vi "Report.vi"(8 "error in":errorcluster, 9 "Received":path, 10 "Approved":path, 11 "Report Nothing in":refnum<class "Report Nothing.lvclass">) -> (0 "error out":errorcluster, 2 "Worked?":bool, 3 "Report Nothing out":refnum<class "Report Nothing.lvclass">)   [LabVIEW 2020, in "Approval Tests.lvlib" / "Report Nothing.lvclass"]
uses:
  Report Nothing.lvclass
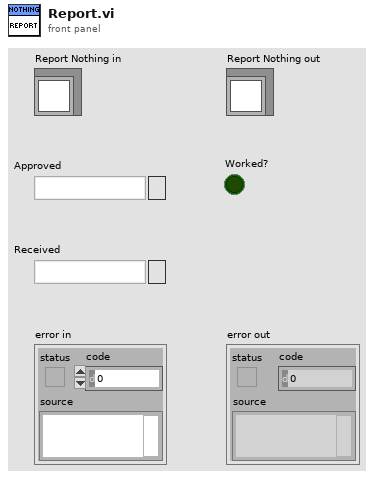
[diagram p1: front panel]
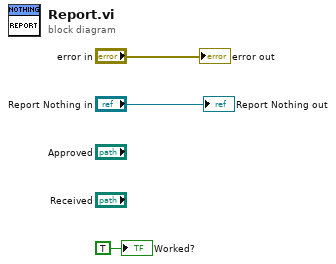
[diagram p0: block diagram]
diagram:
  "error out" <- "error in"
  "Report Nothing out" <- "Report Nothing in"
  "Worked?" <- TRUE ("Reporter Was Launched?")
